vi "image to array.vi"(8 "Path to PNG file":path, 9 "image data":T1, 10 "Normalizare":T2(ring), 11 "Image type":enum16{"Image file (png)", "Image data"}(ring)) -> (0 "Image 28x28":u8[][](graph), 1 "Image 280x280":u8[][](graph), 2 "Image 2d array":dbl[][](array[numeric]), 3 "Image 1d Array":dbl[](array[numeric]), 4 "Nr.pixeli":dbl)   [LabVIEW 2024]
uses:
  <vilib>/picture/picture.llb/imagedata.ctl
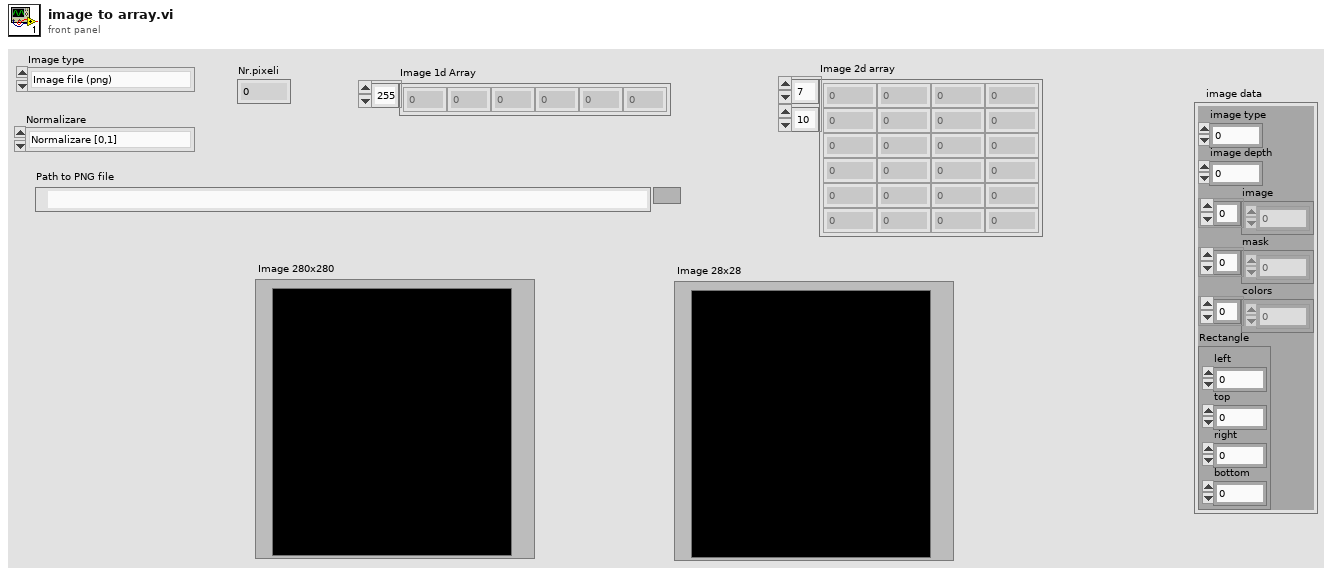
[diagram p1: front panel]
types:
  T1 = typedef "imagedata.ctl" = cluster{"image type":i32, "image depth":i32, "image":u8[], "mask":u8[], "colors":u32[], "Rectangle":cluster{"left":i16, "top":i16, "right":i16, "bottom":i16}}
  T2 = enum16{"Normalizare [0,1]", "Normalizare[-1,1]", "Fara normalizare"}
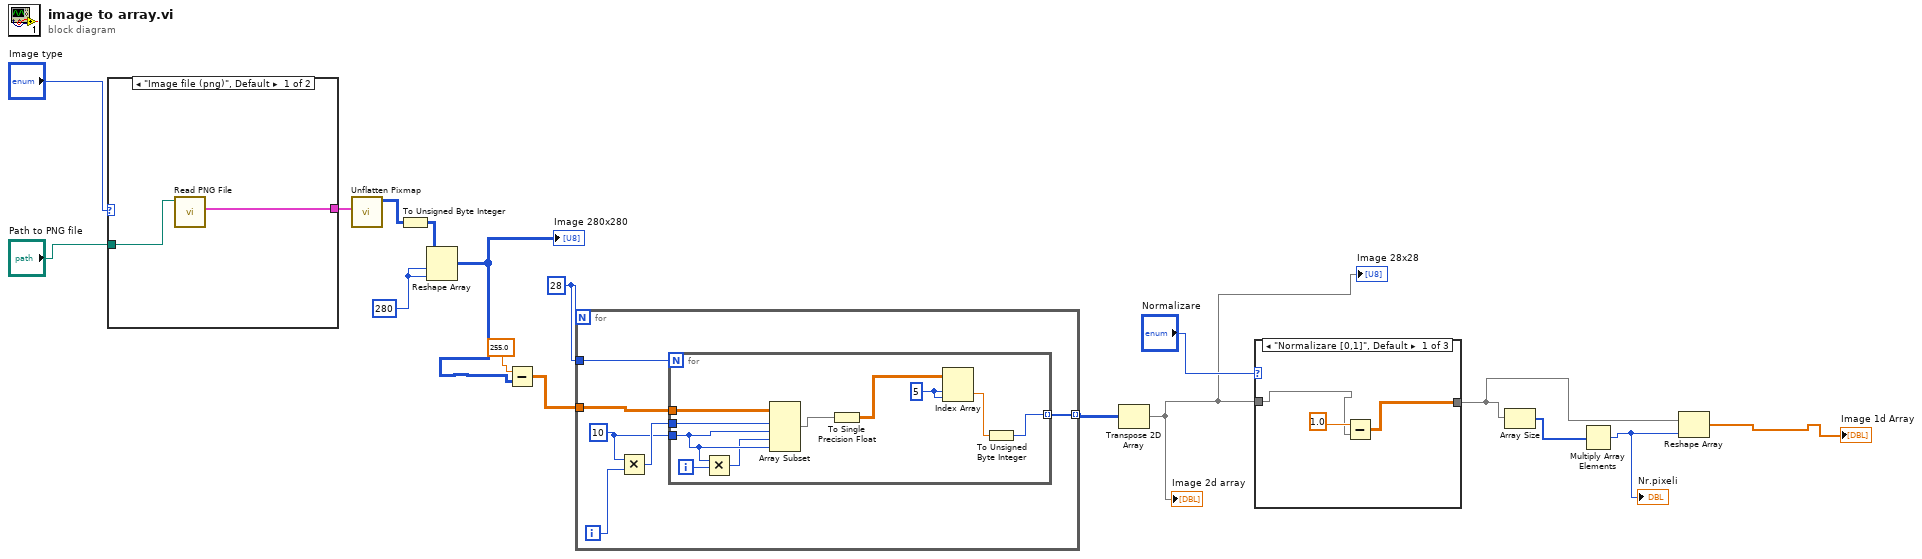
[diagram p0: block diagram]
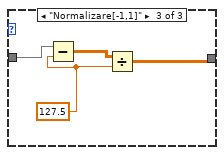
[diagram p3: hidden frame]
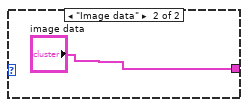
[diagram p4: hidden frame]
diagram:
  w14 = 28
  w15 = 280
  n1 = case shown="\"Image file (png)\", Default" "Image type" {
    tunnel: "Path to PNG file" -> [w19 _]
    tunnel: [w18 "image data"] -> w7
    frame "Image file (png)", Default {
      n2 = call <vilib>:"Read PNG File.vi"("path to PNG file"=w19) -> ("image data"=w18:T1)  [unwired: 8 in, 2 out]
    }
    frame "Image data" {
    }
  }
  n3 = call <vilib>:"Unflatten Pixmap.vi"("image data"=w7) -> ("24-bit pixmap"=w4:u32[][])  [unwired: 4 in, 6 out]
  n4 = To Unsigned Byte Integer(number=w4) -> (unsigned 8bit integer=w3:u8[][])
  n5 = Reshape Array(w3, w15, w15) -> (w5:u8[][])
  "Image 280x280" <- w5
  n6 = Subtract(x=255.0, y=w5) -> (x-y=w6:dbl[][])
  n7 = for {
    N: w14 -> [_]
    tunnel: [w23] -> w13 mode=indexing
    tunnel: w6 -> [w22]
    tunnel: w14 -> [w21]
    i -> [w26]
    w24 = 10
    n8 = Multiply(x=w24, y=w26) -> (x*y=w25:i32)
    n9 = for {
      N: w21 -> [_]
      tunnel: w22 -> [w36]
      tunnel: w25 -> [w35]
      tunnel: w24 -> [w33]
      tunnel: [w30] -> w23 mode=indexing
      i -> [w34]
      w28 = 5
      n10 = Multiply(x=w33, y=w34) -> (x*y=w32:i32)
      n11 = Array Subset(array=w36, index (row)=w35, length (row)=w33, index (col)=w32, length (col)=w33) -> (w31:dbl[][])
      n12 = To Single Precision Float(number=w31) -> (single precision float=w29:sgl[][])
      n13 = Index Array(array=w29, index (row)=w28, index (col)=w28) -> (element=w27:sgl)
      n14 = To Unsigned Byte Integer(number=w27) -> (unsigned 8bit integer=w30:u8)
    }
  }
  n15 = Transpose 2D Array(2D array=w13) -> (transposed array=w2:u8[][])
  "Image 2d array" <- w2
  "Image 28x28" <- w2
  n16 = case shown="\"Normalizare [0,1]\", Default" "Normalizare" {
    tunnel: w2 -> [w38 w40 w44]
    tunnel: [w37 w40 w41] -> w9
    frame "Normalizare [0,1]", Default {
      n17 = Subtract(x=1.0, y=w38) -> (x-y=w37:dbl[][])
    }
    frame "Fara normalizare" {
    }
    frame "Normalizare[-1,1]" {
      w42 = 127.5
      n18 = Subtract(x=w44, y=w42) -> (x-y=w43:dbl[][])
      n19 = Divide(x=w43, y=w42) -> (x/y=w41:dbl[][])
    }
  }
  n20 = Array Size(array=w9) -> (size(s)=w11:i32[])
  n21 = Multiply Array Elements(1:w11) -> (0:w10:i32)
  "Nr.pixeli" <- w10
  n22 = Reshape Array(w9, w10) -> (→"Image 1d Array":dbl[])
